vi "sharp_ir_medium.vi"(11 "ana_volts":dbl) -> (3 "eng_cm":dbl)   [LabVIEW 2012]
panel:
  in  "cm":dbl[](array[numeric])=[100.0, 80.0, 61.0, 40.0, 27.0, 20.0, 15.0, 13.0, 12.0, 9.0, 6.5, 0.0]
  in  "volts":dbl[](array[numeric])=[0.0, 0.4, 0.5, 0.75, 1.0, 1.25, 1.5, 1.75, 2.0, 2.5, 3.0, 5.0]
  # "This function is a transfer function for the Sharp IR GP2Y0A21YK medium range IR rangefinder\nThis curve is copied directly from the Sharp spec sheet transfer curve. Units are cm in that sheet."
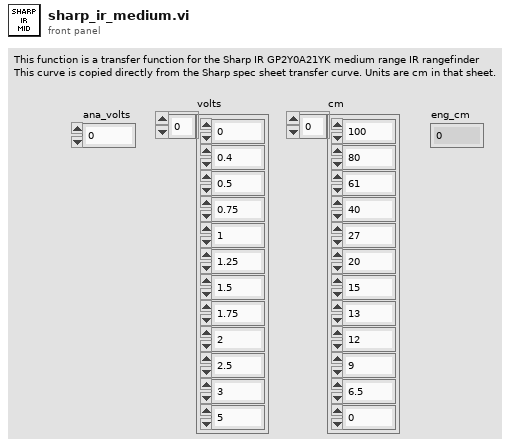
[diagram p1: front panel]
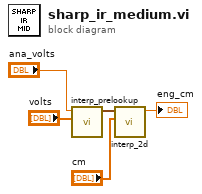
[diagram p0: block diagram]
diagram:
  n1 = call "interp_prelookup.vi"("x"="volts", "X"="ana_volts") -> ("prelookup"=w3:cluster{"frac":dbl, "num":u8})  [unwired: 8 in, 1 out]
  n2 = call "interp_2d.vi"("z"="cm", "prelookup"=w3) -> ("z"=→"eng_cm":dbl)  [unwired: 9 in]
